vi "subGetItemMatchingTarget.vi"(7 "Project ref":refnum<vi>, 8 "error in (no error)":errorcluster, 11 "ProjectItem in":refnum<class "ProjectItem.lvclass">) -> (0 "error out":errorcluster, 2 "TargetItem Ref":refnum<vi>, 3 "ProjectItem out":refnum<class "ProjectItem.lvclass">)   [LabVIEW 2019, in "SolutionBuilder.lvlib" / "ProjectItem.lvclass"]
uses:
  ProjectItem.lvclass
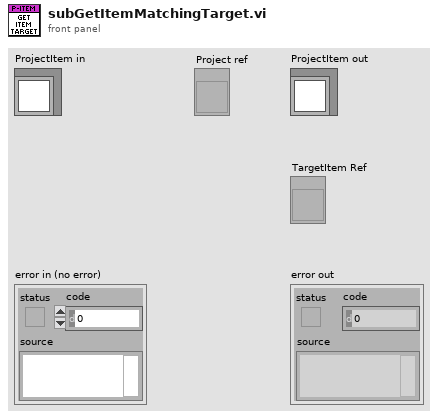
[diagram p1: front panel]
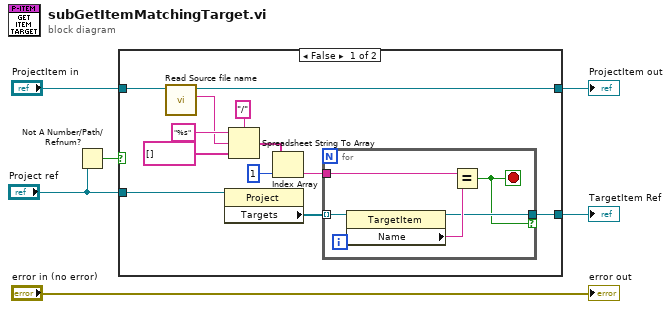
[diagram p0: block diagram]
diagram:
  n1 = Not A Number/Path/Refnum?(number/path/refnum="Project ref") -> (NaN/Path/Refnum?=w1:bool)
  n2 = case shown="False" w1 {
    tunnel: "ProjectItem in" -> [w18 w24]
    tunnel: [w17 w24] -> w4
    tunnel: "Project ref" -> [w10 _]
    tunnel: [w7 _] -> w2
    frame False {
      n3 = call-dynamic "Read Source file name.vi"("ProjectItem in"=w18) -> ("Source file name"=w11:string, "ProjectItem out"=w17:refnum<class "ProjectItem.lvclass">)  [unwired: 9 in]
      n4 = property class="Project"(reference=w10) -> ("Targets"=w9:refnum<vi>[])  [unwired: 1 in, 2 out]
      n5 = Spreadsheet String To Array(delimiter (Tab)="/", format string="%s", spreadsheet string=w11, array type (2D Dbl)=string[] []) -> (array=w13:string[])
      n6 = Index Array(array=w13, index=1) -> (element=w8:string)
      n7 = for {
        tunnel: w9 -> [w23] mode=indexing
        tunnel: w8 -> [w21]
        tunnel: [w20] -> w7 if=w19
        stop <- w19 stop-if-true
        n8 = property class="TargetItem"(reference=w23) -> (reference out=w20:refnum<vi>, "Name"=w22:string)  [unwired: 1 in, 1 out]
        n9 = Equal?(x=w21, y=w22) -> (x = y?=w19:bool)
      }
    }
    frame True {
    }
  }
  "ProjectItem out" <- w4
  "TargetItem Ref" <- w2
  "error out" <- "error in (no error)"
